vi "UI Handler - Download Data.vi"(8 "error in (no error)":errorcluster, 11 "Data Cluster":T1={"Data Display"="", "FP Control Refs"={"Connect to Station Ref"=refnum, "Download Ref"=refnum, "Exit Button Ref"=refnum, "Start Date Refnum"=refnum, "End Date Refnum"=refnum, "Path"=refnum, "COM Port"="", "IP or Phone Ref"=refnum, "TCPIP ID"=refnum, "Reboot Refnum"=refnum, "Datafile Refnum"=refnum}, "FP Indicator Refs"={"Connected Refnum"=refnum, "Data Display Ref"=refnum, "Station ID Ref"=refnum}, "User Events"={"Stop"=refnum, "Update Display"=refnum}, "Message Queues"={"UI"=refnum, "ACQUISITION"=refnum, "PROCESSING"=refnum, "LOGGING"=refnum}, "IS IP?"=FALSE, "Downloading?"=FALSE, "DCP Version"=enum."XPert2", "Processing Loop State"=enum."Get Station  ID", "Username"=refnum, "Password"=refnum}) -> (0 "error out":errorcluster, 3 "Data Cluster out":T1={"Data Display"="", "FP Control Refs"={"Connect to Station Ref"=refnum, "Download Ref"=refnum, "Exit Button Ref"=refnum, "Start Date Refnum"=refnum, "End Date Refnum"=refnum, "Path"=refnum, "COM Port"="", "IP or Phone Ref"=refnum, "TCPIP ID"=refnum, "Reboot Refnum"=refnum, "Datafile Refnum"=refnum}, "FP Indicator Refs"={"Connected Refnum"=refnum, "Data Display Ref"=refnum, "Station ID Ref"=refnum}, "User Events"={"Stop"=refnum, "Update Display"=refnum}, "Message Queues"={"UI"=refnum, "ACQUISITION"=refnum, "PROCESSING"=refnum, "LOGGING"=refnum}, "IS IP?"=FALSE, "Downloading?"=FALSE, "DCP Version"=enum."XPert2", "Processing Loop State"=enum."Get Station  ID", "Username"=refnum, "Password"=refnum})   [LabVIEW 2018]
uses:
  controls/GLDL UI Data.ctl
  controls/Disconnect Control.ctl
  controls/Download Control.ctl
  controls/Exit Control.ctl
  controls/Date Control.ctl
  controls/IP Phone Number Control.ctl
  controls/Reboot Control.ctl
  controls/Connected Indicator.ctl
  controls/Output Indicator.ctl
  controls/Station ID Indicator.ctl
  Message Queue/All Message Queues.ctl
  Message Queue/Message Cluster.ctl
  controls/Processing Loop State.ctl
  Message Queue/Enqueue Message (Single).vi
  Message Queue/GLDL Message Queue.lvlib
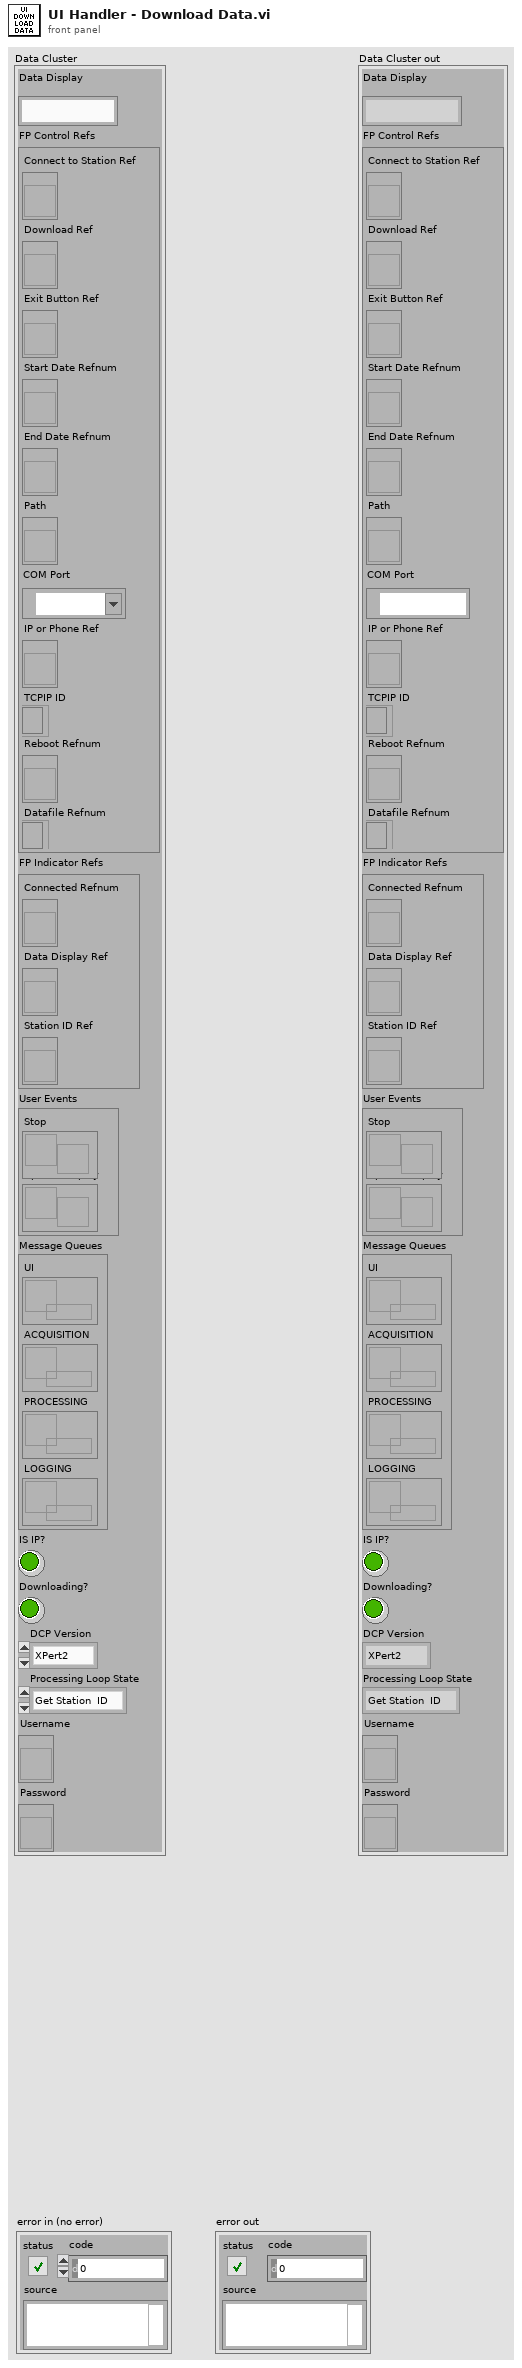
[diagram p1: front panel]
types:
  T1 = typedef "GLDL UI Data.ctl" = cluster{"Data Display":string, "FP Control Refs":cluster{"Connect to Station Ref":refnum<vi>, "Download Ref":refnum<vi>, "Exit Button Ref":refnum<vi>, "Start Date Refnum":refnum<vi>, "End Date Refnum":refnum<vi>, "Path":refnum<vi>, "COM Port":refnum<visa-resource-name>, "IP or Phone Ref":refnum<vi>, "TCPIP ID":refnum<k5>, "Reboot Refnum":refnum<vi>, "Datafile Refnum":refnum<file>}, "FP Indicator Refs":cluster{"Connected Refnum":refnum<vi>, "Data Display Ref":refnum<vi>, "Station ID Ref":refnum<vi>}, "User Events":cluster{"Stop":refnum<user-event>, "Update Display":refnum<user-event>}, "Message Queues":T2, "IS IP?":bool, "Downloading?":bool, "DCP Version":enum16{"XPert", "XPert2"}, "Processing Loop State":T3, "Username":refnum<vi>, "Password":refnum<vi>}
  T2 = typedef "GLDL Message Queue.lvlib/All Message Queues.ctl" = cluster{"UI":refnum<queue>, "ACQUISITION":refnum<queue>, "PROCESSING":refnum<queue>, "LOGGING":refnum<queue>}
  T3 = typedef "Processing Loop State.ctl" = enum16{"Get Station  ID", "Change Directory SD Card", "Change Directory Storage Card", "Downloading", "Idle in DL Directory"}
  T4 = typedef "Date Control.ctl" = timestamp
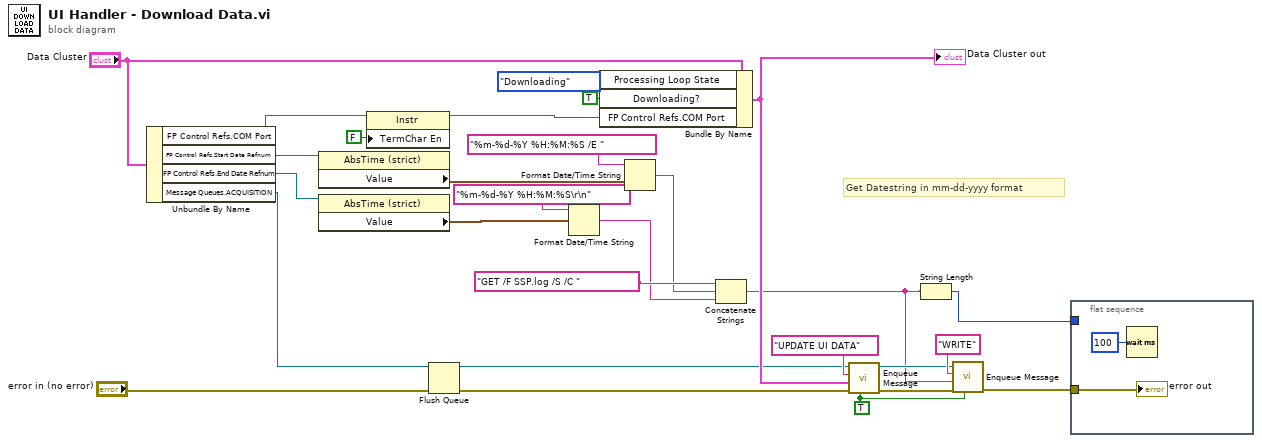
[diagram p0: block diagram]
diagram:
  w10 = TRUE ("Priority Message? (F)")
  # "Get Datestring in mm-dd-yyyy format"
  n1 = Unbundle By Name("Data Cluster") -> ("FP Control Refs.COM Port"=w21:refnum<visa-resource-name>, "FP Control Refs.Start Date Refnum"=w27:refnum<vi>, "FP Control Refs.End Date Refnum"=w8:refnum<vi>, "Message Queues.ACQUISITION"=w9:refnum<queue>)
  n2 = property class="AbsTime (strict)"(reference=w27) -> ("Value"=w24:T4)  [unwired: 1 in, 2 out]
  n3 = property class="AbsTime (strict)"(reference=w8) -> ("Value"=w7:T4)  [unwired: 1 in, 2 out]
  n4 = property class="Instr"(reference=w21, "TermChar En"=FALSE ("Message Based Settings:Termination Character Enable")) -> (reference out=w18:refnum<visa-resource-name>)  [unwired: 1 in, 1 out]
  n5 = Flush Queue(queue=w9, error in (no error)="error in (no error)") -> (queue out=w12:refnum<queue>, error out=w11:errorcluster)  [unwired: 1 out]
  n6 = Format Date/Time String(time format string (%c)="%m-%d-%Y %H:%M:%S\r\n", seconds (now)=w7) -> (date/time string=w5:string)  [unwired: 1 in]
  n7 = Bundle By Name(cluster="Data Cluster", "Processing Loop State"=Processing_Loop_State."Downloading", "Downloading?"=TRUE, "FP Control Refs.COM Port"=w18) -> (w16:T1)
  "Data Cluster out" <- w16
  n8 = Format Date/Time String(time format string (%c)="%m-%d-%Y %H:%M:%S /E ", seconds (now)=w24) -> (date/time string=w22:string)  [unwired: 1 in]
  n9 = Concatenate Strings("GET /F SSP.log /S /C ", w22, w5) -> (w4:string)
  n10 = call-poly "Enqueue Message.vi"("Priority Message? (F)"=w10, "error in (no error)"=w11, "Message Data"=w16, "Message"="UPDATE UI DATA", "Message Queue"=w12) -> ("error out"=w14:errorcluster, "dup Message Queue"=w15:refnum<queue>)  [unwired: 5 in]
  n11 = String Length(string=w4) -> (length=w3:i32)
  n12 = call-poly "Enqueue Message.vi"("Priority Message? (F)"=w10, "error in (no error)"=w14, "Message Data"=w4, "Message"="WRITE", "Message Queue"=w15) -> ("error out"=w23:errorcluster)  [unwired: 5 in, 1 out]
  n13 = flat-sequence {
    tunnel: w23 -> [w30]
    tunnel: w3 -> [_]
    frame #0 {
      n14 = Wait (ms)(milliseconds to wait=u32 100) -> ()  [unwired: 1 out]
      "error out" <- w30
    }
  }
